vi "Singleton Data.vi"(8 "error in":errorcluster, 10 "set? (F)":bool, 11 "Vision Server":refnum<class "Vision Server.lvclass">) -> (0 "error out":errorcluster, 3 "Vision Server Copy":refnum<class "Vision Server.lvclass">)   [LabVIEW 2016, in "Vision Server.lvclass"]
uses:
  Vision Server.lvclass
panel:
  # "This is a global COPY of class data, must be updated \non state changes by server vi"
  # "(better implementation would use DVR)"
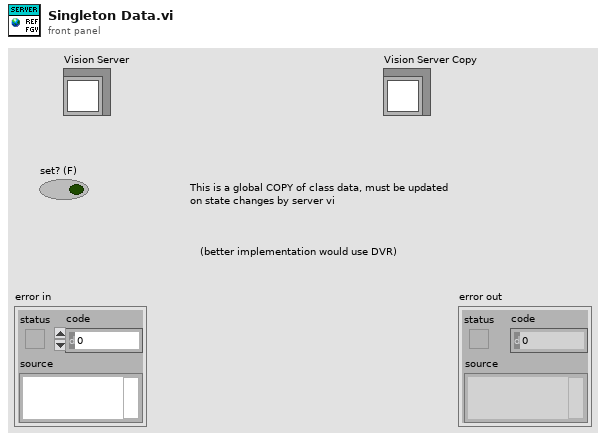
[diagram p1: front panel]
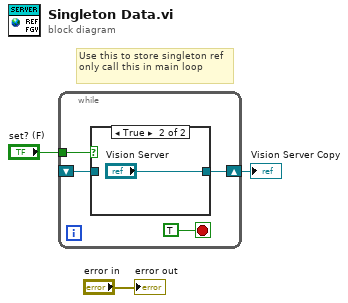
[diagram p0: block diagram]
diagram:
  # "Use this to store singleton ref only call this in main loop"
  n1 = while {
    tunnel: "set? (F)" -> [w7]
    shift-right: [w6] -> w1
    shift-left: _ -> [w5]
    stop <- TRUE stop-if-true
    n2 = case shown="True" w7 {
      tunnel: [w8 "Vision Server"] -> w6
      tunnel: w5 -> [w8 _]
      frame False {
      }
      frame True {
      }
    }
  }
  "Vision Server Copy" <- w1
  "error out" <- "error in"
